vi "Deserialize64.vi"(11 "U64 input":u64) -> (3 "60bit output":bool[](array[boolean]))   [LabVIEW 2012]
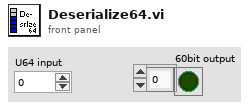
[diagram p1: front panel]
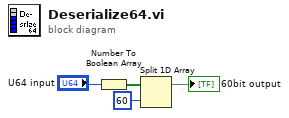
[diagram p0: block diagram]
diagram:
  n1 = Number To Boolean Array(number="U64 input") -> (Boolean array=w3:bool[])
  n2 = Split 1D Array(array=w3, index=60) -> (first subarray=→"60bit output":bool[])  [unwired: 1 out]
